vi "read_bed_position.vi"() -> (0 "Absolute position (pulses)":i32=6040)   [LabVIEW 2019]
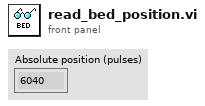
[diagram p1: front panel]
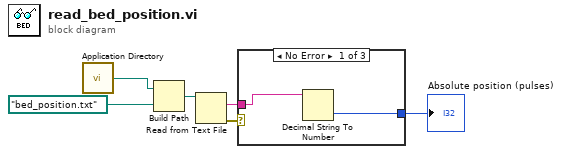
[diagram p0: block diagram]
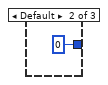
[diagram p2: hidden frame]
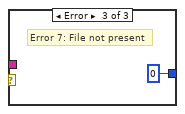
[diagram p3: hidden frame]
diagram:
  n1 = call <vilib>:"Application Directory.vi"() -> ("Application Directory"=w3:path)
  n2 = Build Path(base path=w3, name or relative path=path "bed_position.txt" ("file (use dialog)")) -> (appended path=w4:path)
  n3 = Read from Text File(file (use dialog)=w4) -> (text=w6:string, error out=w5:errorcluster)  [unwired: 3 in, 2 out]
  n4 = case shown="No Error" w5 {
    tunnel: w6 -> [w8 _ _]
    tunnel: [w7 0 0] -> w1
    frame No Error {
      n5 = Decimal String To Number(string=w8) -> (number=w7:i32)  [unwired: 2 in, 1 out]
    }
    frame Default {
    }
    frame Error {
      # "Error 7: File not present"
    }
  }
  "Absolute position (pulses)" <- w1
